vi "Save to file.vi"(8 "error in (no error)":errorcluster, 10 "file path (use dialog)":path, 11 "UserPwd DB in":refnum<class "UserPwd DB.lvclass">) -> (0 "error out":errorcluster, 3 "UserPwd DB out":refnum<class "UserPwd DB.lvclass">)   [LabVIEW 2016, in "UserPwd DB.lvlib" / "UserPwd DB.lvclass"]
uses:
  <userlib>/Common Components/UserPwd DB/UserPwd DB/UserPwd DB.lvclass
  <userlib>/Common Components/UserPwd DB/UserPwd DB/UserPwd DB.lvclass/UserPwd DB.ctl
  <vilib>/addons/_JKI.lib/Serialization/JSON/JKI JSON Serialization.lvlib
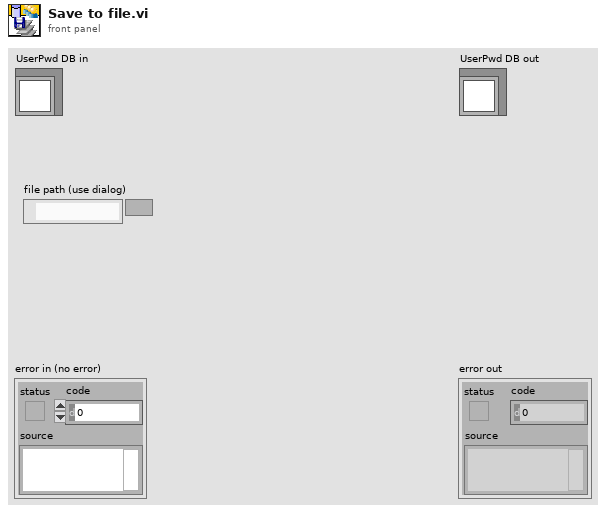
[diagram p1: front panel]
types:
  T1 = enum16{"open", "replace", "create", "open or create", "replace or create", "replace or create with confirmation"}
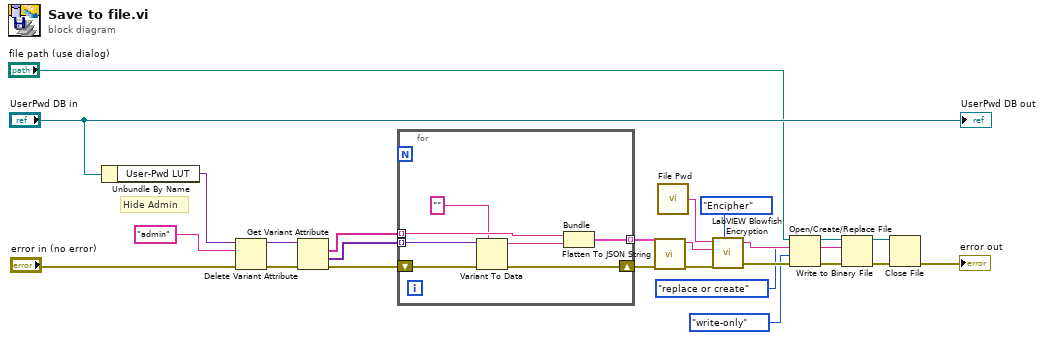
[diagram p0: block diagram]
diagram:
  # "Hide Admin"
  n1 = Unbundle By Name("UserPwd DB in") -> ("User-Pwd LUT"=w22:variant)
  n2 = Delete Variant Attribute(4:"error in (no error)", 6:"admin" ("name (all attributes)"), 7:w22) -> (0:w23:errorcluster, 3:w21:variant)  [unwired: 1 out]
  n3 = Get Variant Attribute(Variant=w21, error in=w23) -> (names=w17:string[], values=w24:variant[], error out=w25:errorcluster)  [unwired: 2 in, 1 out]
  n4 = for {
    shift-right: [w31] -> w16
    shift-left: w25 -> [w32]
    tunnel: w24 -> [w30] mode=indexing
    tunnel: w17 -> [w29] mode=indexing
    tunnel: [w27] -> w15 mode=indexing
    n5 = Variant To Data(error in=w32, type="", Variant=w30) -> (data=w28:string, error out=w31:errorcluster)
    n6 = Bundle(w29, w28) -> (w27:cluster{string, string})  [unwired: 1 in]
  }
  n7 = call <vilib>:"Flatten To JSON String.vi"("error in (no error)"=w16, "Variant"=w15) -> ("error out"=w14:errorcluster, "JSON String"=w12:string)  [unwired: 8 in]
  n8 = call <userlib>:"File Pwd.vi"() -> ("String"=w13:string)
  n9 = call <userlib>:"LabVIEW Blowfish Encryption.vi"("Password"=w13, "Enc/Dec"=enum16{"Encipher", "Decipher"}."Encipher", "Input Text"=w12, "error in (no error)"=w14) -> ("Output text"=w9:string, "error out"=w10:errorcluster)  [unwired: 2 in, 1 out]
  n10 = Open/Create/Replace File(file path (use dialog)="file path (use dialog)", error in=w10, operation (0:open)=T1."replace or create", access (0:read/write)=enum16{"read/write", "read-only", "write-only"}."write-only") -> (refnum out=w3:refnum<file>, error out=w7:errorcluster)  [unwired: 2 in, 1 out]
  n11 = Write to Binary File(file (use dialog)=w3, data=w9, error in=w7) -> (refnum out=w1:refnum<file>, error out=w8:errorcluster)  [unwired: 3 in, 1 out]
  n12 = Close File(refnum=w1, error in=w8) -> (error out=→"error out":errorcluster)  [unwired: 1 out]
  "UserPwd DB out" <- "UserPwd DB in"
